vi "TestRead Infrared Sensor.vi"() -> ()   [LabVIEW 2020]
uses:
  <vilib>/High Genius/HG_WSI_Tookit/Dependencies/Library/Analog In/Analog In.lvclass
  C:/Program Files (x86)/National Instruments/LabVIEW 2020/vi.lib/High Genius/HG_WSI_Tookit/Dependencies/Library/HG_LIB/HG_LIB.lvclass
  <vilib>/Platform/TimedLoop/XDataNode/timing_clust.ctl
  <vilib>/Platform/TimedLoop/XDataNode/nitl_modes.ctl
  <vilib>/Platform/TimedLoop/XDataNode/wakeup.ctl
  <vilib>/Platform/TimedLoop/XDataNode/XDataNode.xnode
  <vilib>/High Genius/HG_WSI_Tookit/Dependencies/Library/HG_LIB/HG_LIB.lvclass
  <vilib>/Platform/TimedLoop/XDataNode/XDNodeRunTimeDep.lvlib
panel:
  out "IR Right":dbl
  out "IR Left":dbl
  in  "stop":bool
  # "Control Description:\n1. IR: infrared ranging sensor on the right side of robot\n\nDescription of operation procedure steps:\n1. Running program\n2. Move the object in front of the infrared sensor and observe the distance of the infrared sensor data display."
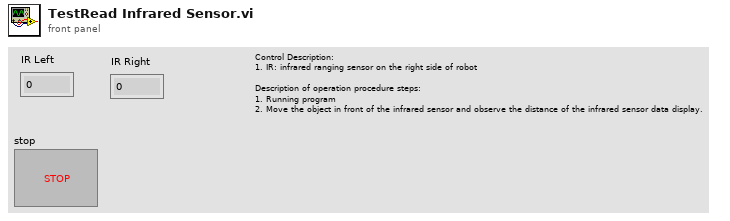
[diagram p1: front panel]
types:
  T1 = enum16{"DI", "DO", "AI", "Pulse", "PWM", "ISQ", "ENC", "CAN", "IIC", "IMU"}
  T2 = enum16{"0", "1", "2", "3", "4", "5", "6", "7", "8", "9", "10", "11", "12", "13", "14", "15", "16", "17", "18", "19", "20", "21", "22", "23", "24", "25"}
  T3 = typedef "XDNodeRunTimeDep.lvlib/timing_clust.ctl" = cluster{"Expected End [f-1]":u64, "Actual End [f-1]":u64, "Finished Late? [f-1]":bool, "Expected End [i-1]":u64, "Actual End [i-1]":u64, "Finished Late? [i-1]":bool, "Expected Start [i]":u64, "Actual Start [i]":u64, "Expected Start [f]":u64, "Actual Start [f]":u64, "Source Name":string, "Structure Name":string, "Period":i64, "Deadline":i64, "Offset":i64, "Start":i64, "Priority":i32, "Timeout":i32, "Mode":T4, "Wakeup Reason":T5, "Error":errorcluster, "Source Type":string, "Secondary Source Type":string, "Global End Time":u64, "Global Start Time":u64, "Frame Duration":u64, "Iteration Duration":u64, "Assigned CPU":i32, "I/O Scan Engine Mode":u32}
  T4 = typedef "XDNodeRunTimeDep.lvlib/nitl_modes.ctl" = enum32{"No Change", "Process missed periods, maintain original phase", "Discard missed periods, maintain original phase", "Process missed periods, ignore original phase", "Discard missed periods, ignore original phase"}
  T5 = typedef "XDNodeRunTimeDep.lvlib/wakeup.ctl" = enum32{"Normal", "Aborted", "Asynchronous wakeup", "Timing source error", "Timed loop error", "Timeout"}
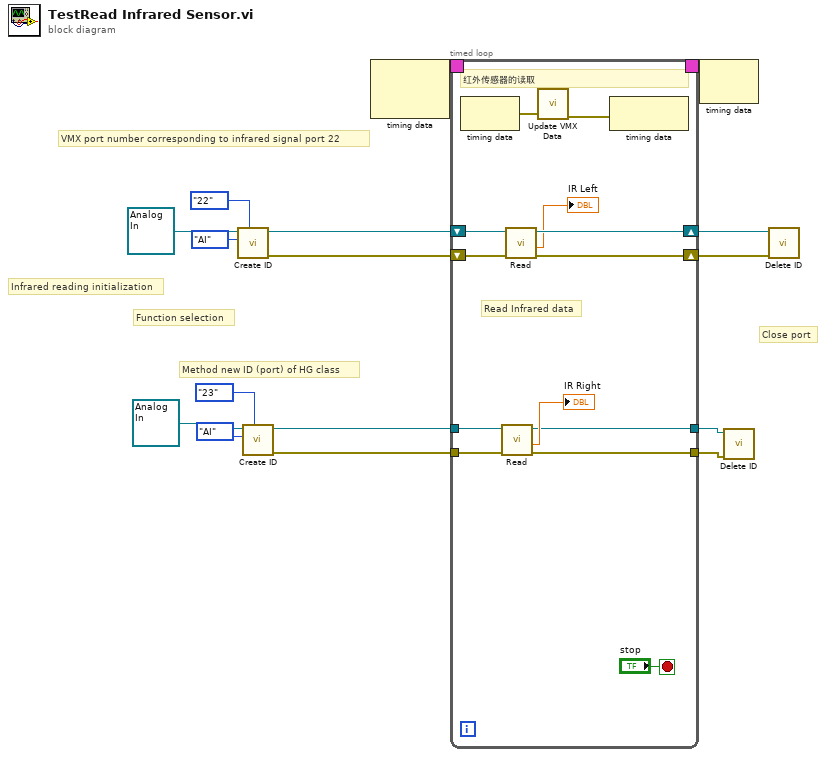
[diagram p0: block diagram]
diagram:
  # "Close port"
  # "Method new ID (port) of HG class"
  # "Function selection"
  # "Infrared reading initialization"
  # "VMX port number corresponding to infrared signal port 22"
  n1 = call <vilib>:"Create ID.vi"("NO"=T2."22", "Function"=T1."AI", "HG_LIB in"=refnum<class "Analog In.lvclass"> refnum ("Analog In.lvclass")) -> ("error out"=w14:errorcluster, "HG_LIB out"=w10:refnum<class "Analog In.lvclass">)  [unwired: 7 in]
  n2 = call <vilib>:"Create ID.vi"("NO"=T2."23", "Function"=T1."AI", "HG_LIB in"=refnum<class "Analog In.lvclass"> refnum ("Analog In.lvclass")) -> ("error out"=w3:errorcluster, "HG_LIB out"=w4:refnum<class "Analog In.lvclass">)  [unwired: 7 in]
  n3 = node-c288() -> (w16:T3)  [unwired: 2 in]
  n4 = timed-loop {
    shift-right: [w27] -> w12
    shift-left: w14 -> [w29]
    shift-right: [w28] -> w13
    shift-left: w10 -> [w26]
    timing: w16 -> [_]
    timing-out: [_] -> w15
    tunnel: w4 -> [w21]
    tunnel: w3 -> [w20]
    tunnel: [w18] -> w2
    tunnel: [w17] -> w1
    stop <- "stop" stop-if-true
    # "Read Infrared data"
    # "红外传感器的读取"
    n5 = node-c288() -> (w24:errorcluster)  [unwired: 1 in]
    n6 = call <vilib>:"Read.vi"("error in (no error)"=w20, "Analog In in"=w21) -> ("error out"=w17:errorcluster, "IR"=→"IR Right":dbl, "Analog In out"=w18:refnum<class "Analog In.lvclass">)  [unwired: 6 in, 1 out]
    n7 = call <vilib>:"Read.vi"("error in (no error)"=w29, "Analog In in"=w26) -> ("error out"=w27:errorcluster, "IR"=→"IR Left":dbl, "Analog In out"=w28:refnum<class "Analog In.lvclass">)  [unwired: 6 in, 1 out]
    n8 = call <vilib>:"Update VMX Data.vi"("error in (no error)"=w24) -> ("error out"=w23:errorcluster)  [unwired: 10 in]
    n9 = node-c288(w23) -> ()  [unwired: 1 out]
  }
  n10 = node-c288(w15) -> ()  [unwired: 1 out]
  n11 = call <vilib>:"Delete ID.vi"("error in (no error)"=w1, "HG_LIB in"=w2) -> ()  [unwired: 8 in, 2 out]
  n12 = call <vilib>:"Delete ID.vi"("error in (no error)"=w12, "HG_LIB in"=w13) -> ()  [unwired: 8 in, 2 out]
